vi "Gui_Fill_Ring_From_File.vi"(8 "error in (no error)":errorcluster, 9 "Resource Name":string="Users.txt", 10 "Resource Path":path=path "D:/S.O.F.T.S/LABVIEW/PIL/resources", 11 "Refnum ChneDér":refnum<vi>) -> (0 "error out":errorcluster, 1 "Refnum ChneDér 2":refnum<vi>, 2 "Table":string[](array[string]), 3 "Text":string)   [LabVIEW 2015]
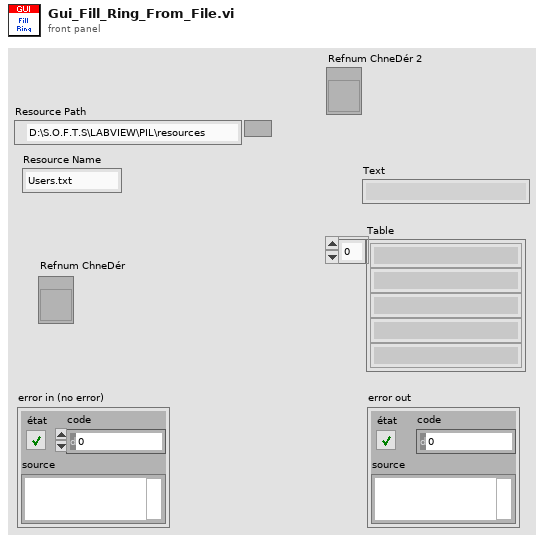
[diagram p1: front panel]
types:
  T1 = enum16{"open", "replace", "create", "open or create", "replace or create", "replace or create with confirmation"}
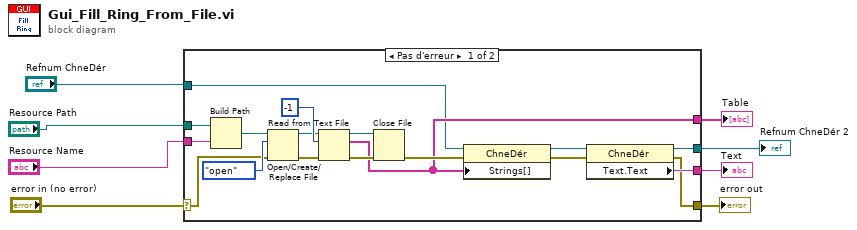
[diagram p0: block diagram]
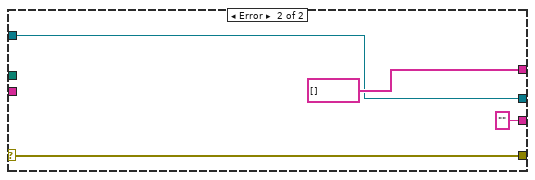
[diagram p2: hidden frame]
diagram:
  n1 = case shown="Pas d'erreur" "error in (no error)" {
    selector: "error in (no error)" -> [w15 w30]
    tunnel: "Resource Path" -> [w26 _]
    tunnel: "Resource Name" -> [w25 _]
    tunnel: [w16 string[] []] -> w4
    tunnel: [w11 w30] -> w5
    tunnel: [w12 "" ("Text.Text")] -> w3
    tunnel: "Refnum ChneDér" -> [w10 w27]
    tunnel: [w9 w27] -> w1
    frame No Error {
      n2 = Build Path(base path=w26, name or relative path=w25) -> (appended path=w22:path)
      n3 = Open/Create/Replace File ("Ouvrir/Créer/Remplacer un fichier")(file path (use dialog)=w22, error in=w15, operation (0:open)=T1."open") -> (refnum out=w23:refnum<file>, error out=w20:errorcluster)  [unwired: 3 in, 1 out]
      n4 = Read from Text File ("Lire un fichier texte")(file (use dialog)=w23, count=-1 ("nombre"), error in=w20) -> (refnum out=w18:refnum<file>, text=w16:string[], error out=w19:errorcluster)  [unwired: 1 in, 1 out]
      n5 = Close File(refnum=w18, error in=w19) -> (error out=w17:errorcluster)  [unwired: 1 out]
      n6 = property class="ChneDér"(reference=w10, error in=w17, "Strings[]"=w16) -> (reference out=w14:refnum<vi>, error out=w13:errorcluster)
      n7 = property class="ChneDér"(reference=w14, error in=w13) -> (reference out=w9:refnum<vi>, error out=w11:errorcluster, "Text.Text"=w12:string)
    }
    frame Error {
    }
  }
  "Table" <- w4
  "error out" <- w5
  "Text" <- w3
  "Refnum ChneDér 2" <- w1
